vi "TCE_Config.vi"(11 "Cluster":T1={"Core"={"Current VI Reference"=refnum, "Close Panel on Exit?"=FALSE}, "Image Out"=refnum, "State"=0, "Points"={"Top Left"={"X"=0.0, "Y"=0.0}, "Top Right"={"X"=0.0, "Y"=0.0}, "Bottom Left"={"X"=0.0, "Y"=0.0}, "Bottom Right"={"X"=0.0, "Y"=0.0}, "x space 2"=0.0, "y space 2"=0.0, "x_space"=0.0, "y_space"=0.0, "Pixels"=[], "Fixpoint"={"X"=0.0, "Y"=0.0}}, "img_array"=[], "Temps"=[], "Temps_Array"=[], "Scan Area"=0.0, "Fixpoint Area"=0.0, "Config"={"Freezing"={"Cutoff"=2.0, "EndIndex"=2}}, "PCR Size"=0, "ImageCount"=0, "ShowGradient"=FALSE} {"Points"."Bottom Right"."Y" format="%.2f"; "Points"."Bottom Right"."X" format="%.2f"; "Points"."Top Left"."Y" format="%.2f"; "Points"."Top Left"."X" format="%.2f"; "Points"."Top Right"."Y" format="%.2f"; "Points"."Top Right"."X" format="%.2f"; "Points"."Bottom Left"."Y" format="%.2f"; "Points"."Bottom Left"."X" format="%.2f"; "Points"."Fixpoint"."Y" format="%.2f"; "Points"."Fixpoint"."X" format="%.2f"}) -> (0 "Canceled":bool, 3 "Config out":T1={"Core"={"Current VI Reference"=refnum, "Close Panel on Exit?"=FALSE}, "Image Out"=refnum, "State"=0, "Points"={"Top Left"={"X"=0.0, "Y"=0.0}, "Top Right"={"X"=0.0, "Y"=0.0}, "Bottom Left"={"X"=0.0, "Y"=0.0}, "Bottom Right"={"X"=0.0, "Y"=0.0}, "x space 2"=0.0, "y space 2"=0.0, "x_space"=0.0, "y_space"=0.0, "Pixels"=[], "Fixpoint"={"X"=0.0, "Y"=0.0}}, "img_array"=[], "Temps"=[], "Temps_Array"=[], "Scan Area"=0.0, "Fixpoint Area"=0.0, "Config"={"Freezing"={"Cutoff"=2.0, "EndIndex"=2}}, "PCR Size"=0, "ImageCount"=0, "ShowGradient"=FALSE} {"Points"."Bottom Right"."Y" format="%.2f"; "Points"."Bottom Right"."X" format="%.2f"; "Points"."Top Left"."Y" format="%.2f"; "Points"."Top Left"."X" format="%.2f"; "Points"."Top Right"."Y" format="%.2f"; "Points"."Top Right"."X" format="%.2f"; "Points"."Bottom Left"."Y" format="%.2f"; "Points"."Bottom Left"."X" format="%.2f"; "Points"."Fixpoint"."Y" format="%.2f"; "Points"."Fixpoint"."X" format="%.2f"})   [LabVIEW 2022 SP3]
uses:
  DataCluster_TCAL.ctl
  <vilib>/vision/Image Controls.llb/IMAQ Image.ctl
  TCE_Config.ctl
panel:
  out "Tutorial":string="Gradients larger than (std.dev × Cutoff) are determined as freezing points.\n\nReducing cutoff allows for smaller gradient freezing to be detected.\n\nNote: Too low cutoff can cause false positive freezing calculations. "
  in  "freezeCutoff":dbl=2.0 caption="Freezing Cutoff" min=1.0 max=100.0 format="%.2g"
  in  "OK":bool
  in  "Cancel":bool
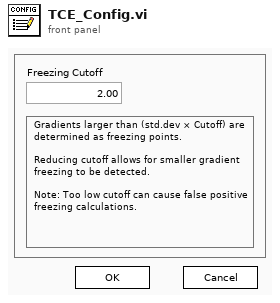
[diagram p1: front panel]
types:
  T1 = typedef "DataCluster_TCAL.ctl" = cluster{"Core":cluster{"Current VI Reference":refnum<vi>, "Close Panel on Exit?":bool}, "Image Out":T2, "State":i32, "Points":cluster{"Top Left":T3, "Top Right":T3, "Bottom Left":T3, "Bottom Right":T3, "x space 2":dbl, "y space 2":sgl, "x_space":sgl, "y_space":sgl, "Pixels":cluster{"X":i32, "Y":i32}[][], "Fixpoint":T3}, "img_array":T2[], "Temps":dbl[], "Temps_Array":dbl[][], "Scan Area":dbl, "Fixpoint Area":dbl, "Config":T4, "PCR Size":u16, "ImageCount":i32, "ShowGradient":bool}
  T2 = typedef "IMAQ Image.ctl" = refnum<image>
  T3 = typedef "IMAQ Point" = cluster{"X":sgl, "Y":sgl}
  T4 = typedef "TCE_Config.ctl" = cluster{"Freezing":cluster{"Cutoff":dbl, "EndIndex":i32}}
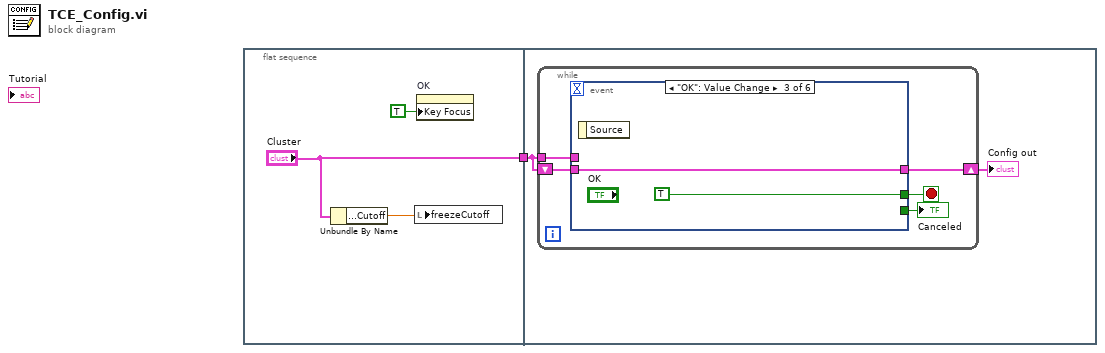
[diagram p0: block diagram]
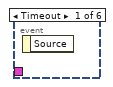
[diagram p2: hidden frame]
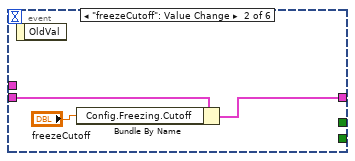
[diagram p3: hidden frame]
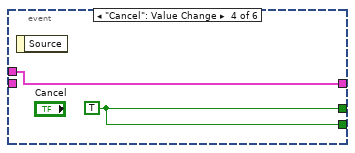
[diagram p4: hidden frame]
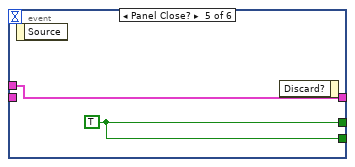
[diagram p5: hidden frame]
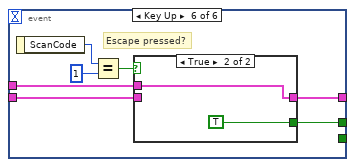
[diagram p6: hidden frame]
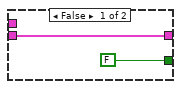
[diagram p7: hidden frame]
diagram:
  n1 = flat-sequence {
    tunnel: ["Cluster"] -> w1
    tunnel: w1 -> [w6]
    frame #0 {
      n2 = Unbundle By Name("Cluster") -> ("Config.Freezing.Cutoff"=w2:dbl)
      n3 = local write "freezeCutoff"(w2) -> ()
      n4 = property on="OK" class="Bool"("Key Focus"=TRUE) -> ()  [unwired: 2 in, 2 out]
    }
    frame #1 {
      n5 = while {
        shift-right: [w11] -> w5
        shift-left: w6 -> [w10]
        tunnel: w6 -> [w9]
        stop <- w8 stop-if-true
        n6 = event shown="[2] \"OK\": Value Change" {
          selector: _ -> [_ _ _ _ _ _]
          dyn-events: _ -> [_ _ _ _ _ _]
          timeout: _ -> [_ _ _ _ _ _]
          tunnel: w10 -> [_ w14 w16 _ _ w21]
          tunnel: [_ w13 w16 w18 w20 w23] -> w11
          tunnel: w9 -> [_ _ _ w18 w20 w22]
          tunnel: [_ _ TRUE w17 w19 w27] -> w8
          tunnel: [_ _ _ w17 w19 _] -> w7
          event Timeout {
            n7 = event-data() -> ()  [unwired: 1 in, 1 out]
          }
          event "freezeCutoff": Value Change {
            n8 = event-data() -> ()  [unwired: 1 in, 1 out]
            n9 = Bundle By Name(cluster=w14, "Config.Freezing.Cutoff"="freezeCutoff") -> (w13:T1)
          }
          event "OK": Value Change {
            n10 = event-data() -> ()  [unwired: 1 in, 1 out]
          }
          event "Cancel": Value Change {
            w17 = TRUE
            n11 = event-data() -> ()  [unwired: 1 in, 1 out]
          }
          event Panel Close? {
            w19 = TRUE
            n12 = event-data() -> ()  [unwired: 1 in, 1 out]
            n13 = event-data() -> ()  [unwired: 2 in, 1 out]
          }
          event Key Up {
            # "Escape pressed?"
            n14 = event-data() -> ("ScanCode"=w26:i16)  [unwired: 1 in]
            n15 = Equal?(x=w26, y=i16 1) -> (x = y?=w24:bool)
            n16 = case shown="True" w24 {
              tunnel: [FALSE TRUE] -> w27
              tunnel: [w29 w30] -> w23
              tunnel: w22 -> [_ w30]
              tunnel: w21 -> [w29 _]
              frame False {
              }
              frame True {
              }
            }
          }
        }
        "Canceled" <- w7
      }
      "Config out" <- w5
    }
  }
